vi "main.vi"() -> ()   [LabVIEW 2009]
uses:
  subvi/activity_info.vi
  <vilib>/Utility/file.llb/Write To Spreadsheet File (DBL).vi
panel:
  in  "Slide":cluster{dbl, dbl}(slide) scale=0.0..1.0
  out "above threshold":dbl(slide) scale=0.0..1.0
  in  "Threshold":dbl(slide)=0.85 scale=0.0..1.0
  out "Correlations":dbl[](graph)
  out "Analyzing":u8(slide) scale=0.0..100.0
  in  "analyze correlations":bool
  in  "Reference Signal":i32
  in  "Reference Signals":dbl[][](array[numeric])
  in  "Save Signal":bool
  in  "read weights":bool
  out "max amplitude":dbl(slide) scale=0.0..2.0
  in  "Path":path=path "E:/Sensor/data/Craig walking ADI.csv"
  out "C":bool
  out "B":bool
  out "A":bool
  in  "write data":bool
  out "Fundamental frequency":dbl(slide) scale=0.0..6.0
  in  "Normalize":bool
  out "high":bool
  out "med":bool
  out "low":bool
  out "RMS":dbl(slide) scale=0.0..10.0
  in  "write to memory":bool
  out "activity output":u16(ring) items=["A", "B", "C", "D"]
  out "output":dbl[](array[slide]) scale=0.0..1.0
  in  "stop learning":bool
  out "Error (training)":dbl(graph)
  in  "Learning Rate":dbl(slide)=0.336734693877551 scale=0.0..1.0
  in  "Beta":dbl(slide)=1.0 scale=0.0..1.0
  in  "train":bool
  in  "Number of hidden neurons":i32(slide)=9 scale=0.0..20.0
  in  "delete state":bool
  in  "state":u32
  in  "activity":u16(ring) items=["A", "B", "C", "D", "E", "F", "G", "H"]
  in  "save state":bool
  in  "Tab Control":T1(tab)=enum."FFT on data 1"
  out "Time data on X',Y',Z'":T2(graph)
  out "FFT on X',Y',Z'":T3(graph)
  out "Filtered signal":dbl[](graph)
  out "Magnitude of time data":cluster{dbl[], dbl[]}(graph)
  out "activity states":T4(graph)
  in  "Sensor":u16(ring) items=["Sensor 1", "Sensor 2", "Sensor 3"]
  in  "Sensor Type":u16(ring) items=["Acceleration", "Rotation"]
  in  "Sensor Brand 1":u16(ring) items=["ADXL", "Kinetisense"]
  in  "End time (s) 1":dbl(slide)=10.0 scale=0.0..200.0
  in  "FFT interval (s) 1":dbl(slide)=4.0 scale=0.0..40.0
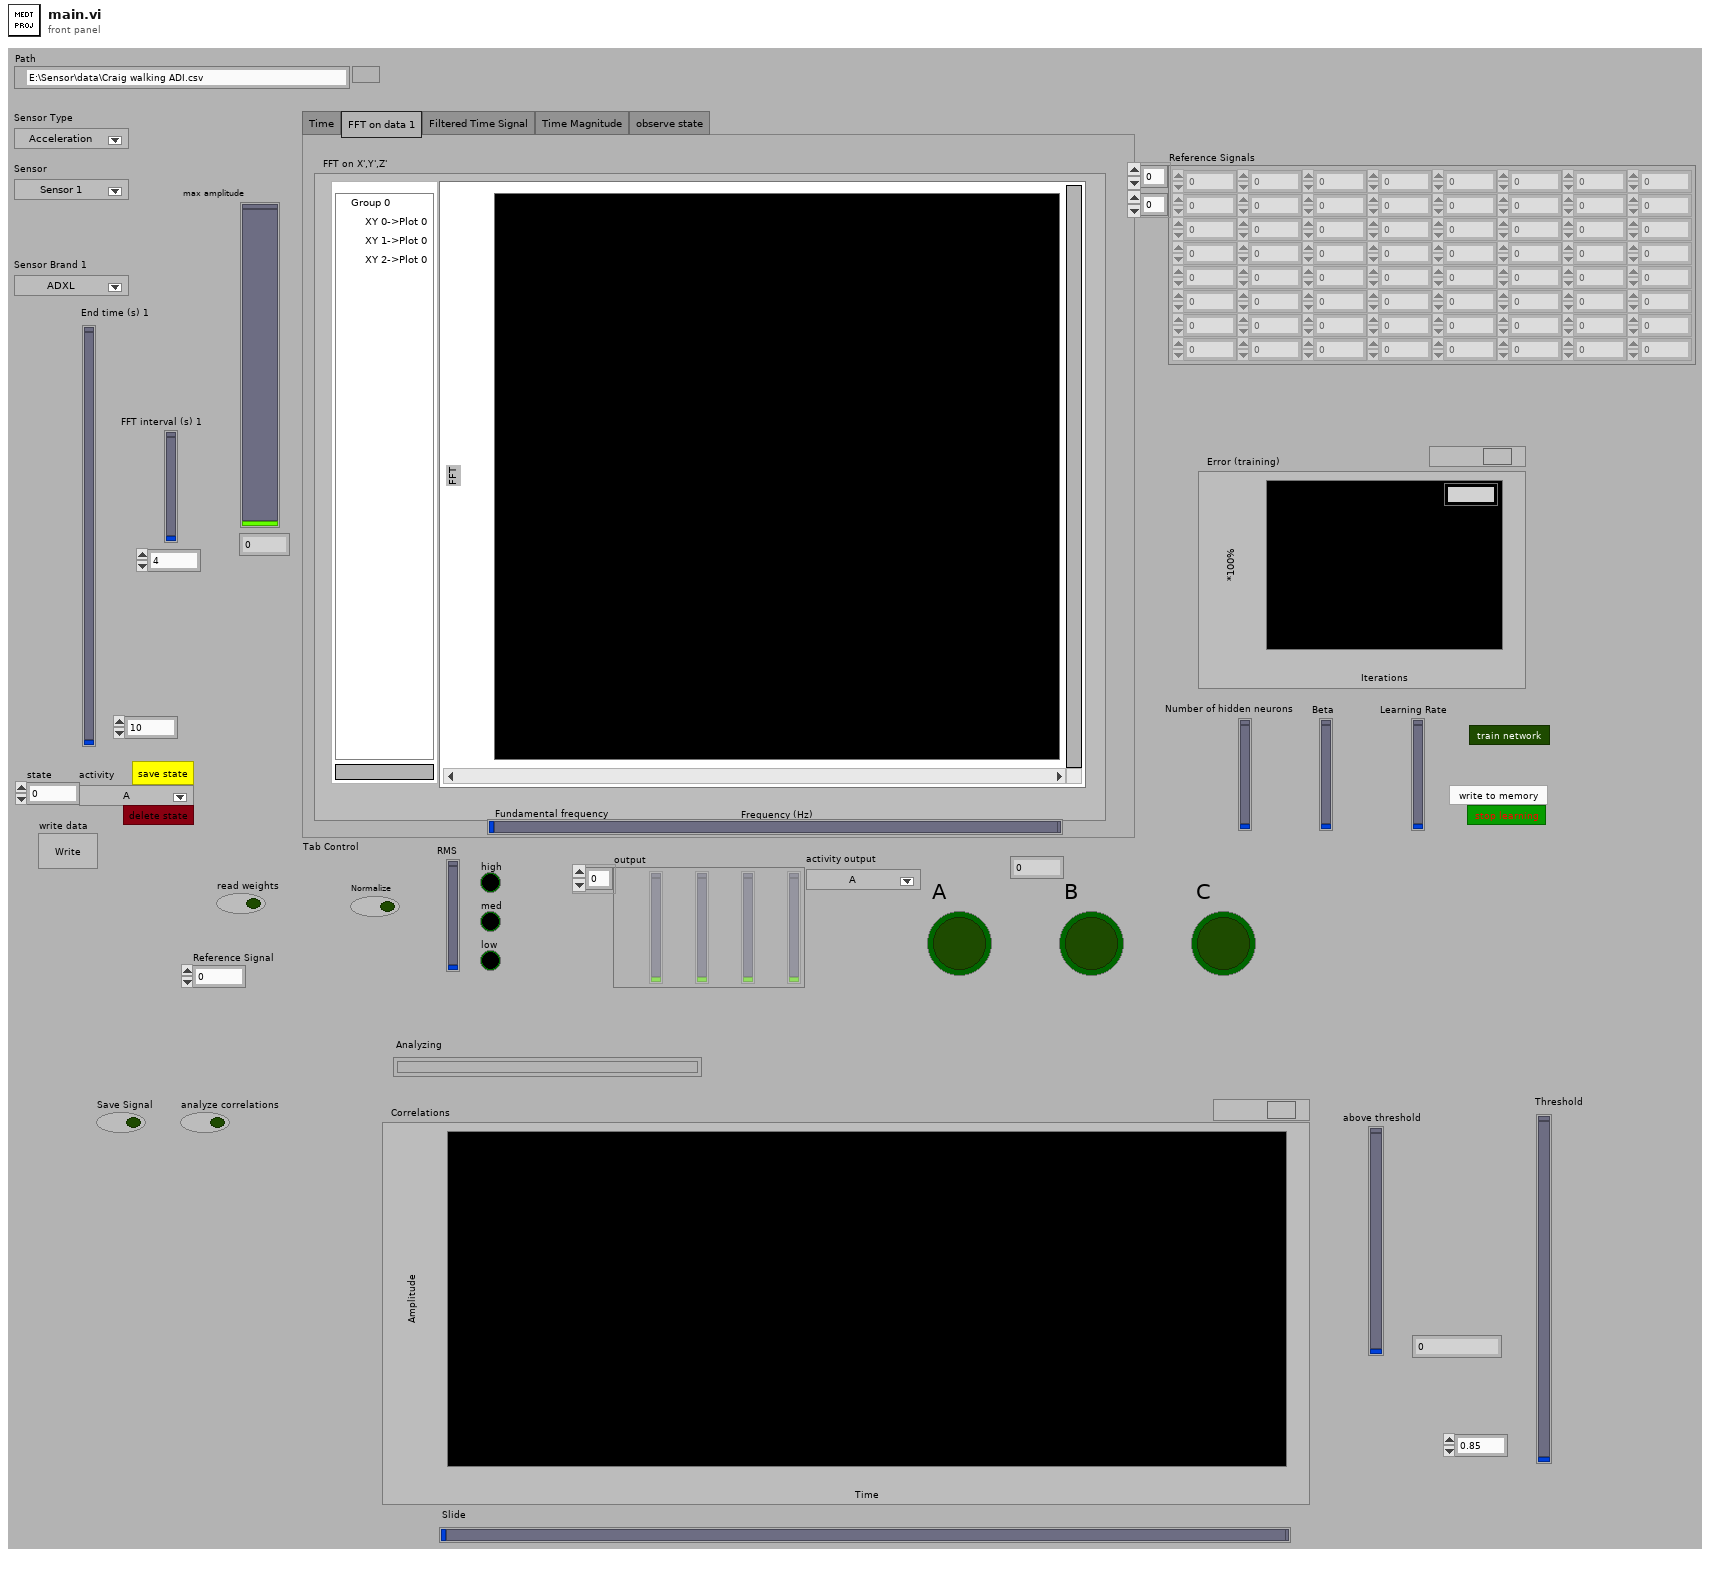
[diagram p1: front panel]
types:
  T1 = enum32{"Time", "FFT on data 1", "Filtered Time Signal", "Time Magnitude", "observe state"}
  T2 = cluster{cluster{dbl[], "Data out":dbl[]}, cluster{dbl[], "Data out":dbl[]}, cluster{dbl[], "Data out":dbl[]}}
  T3 = cluster{"XY Graph":cluster{dbl[], "magnitude":dbl[]}, "XY Graph":cluster{dbl[], "magnitude":dbl[]}, "XY Graph":cluster{dbl[], "magnitude":dbl[]}}
  T4 = cluster{cluster{dbl[], "Bicycling":dbl[]}, cluster{dbl[], "Bicycling":dbl[]}, cluster{dbl[], dbl[]}, cluster{dbl[], dbl[]}, cluster{dbl[], dbl[]}}
  T5 = cluster{"activity":u16, "save state":bool, "state":u32, bool, "peaks":dbl[][], bool}
  T6 = cluster{"activity":u16, "save state":bool, "state":u32, bool, "peaks":dbl[][], "write to memory":bool}
  T7 = cluster{"A":dbl[][], "B":dbl[][], "C":dbl[][], "D":dbl[][], "E":dbl[][], "F":dbl[][], "G":dbl[][], "H":dbl[][]}
  T8 = cluster{cluster{dbl[], dbl[]}, cluster{dbl[], dbl[]}, cluster{dbl[], dbl[]}}
  T9 = cluster{"Cluster":cluster{dbl[], "activity":dbl[]}, "Cluster":cluster{dbl[], "activity":dbl[]}, cluster{dbl[], dbl[]}, cluster{dbl[], dbl[]}, cluster{dbl[], dbl[]}}
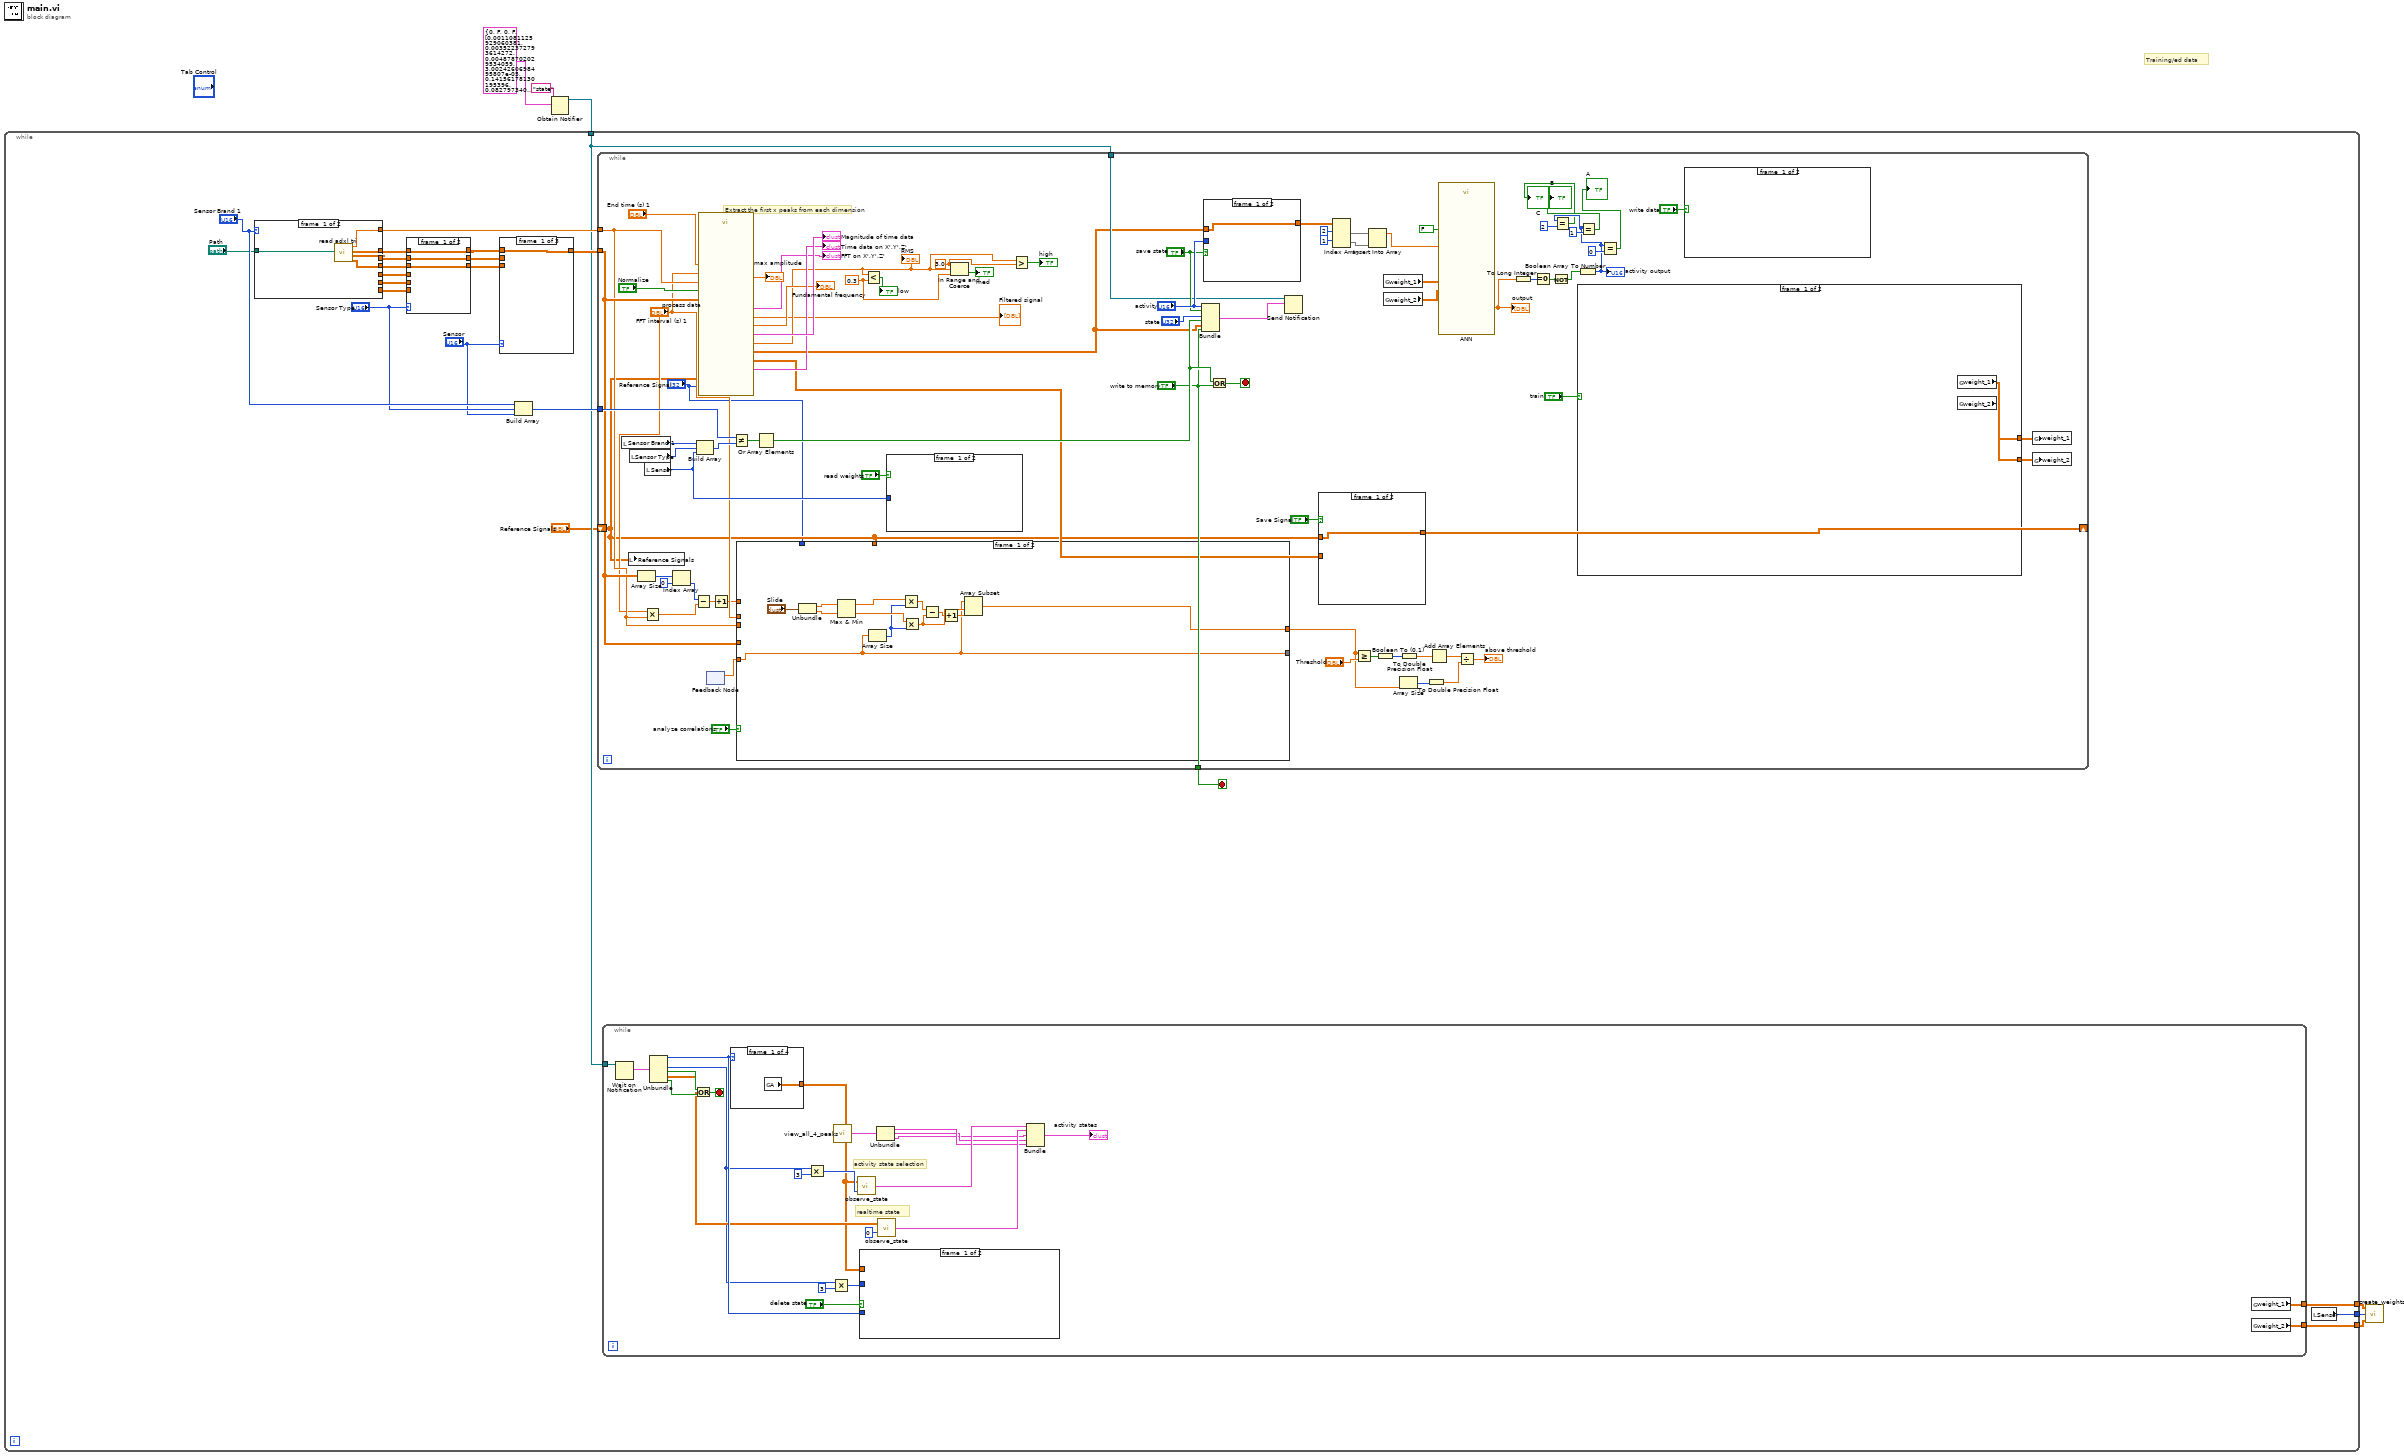
[diagram p0: block diagram]
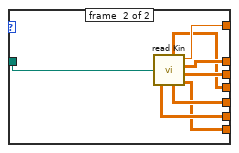
[diagram p5: hidden frame]
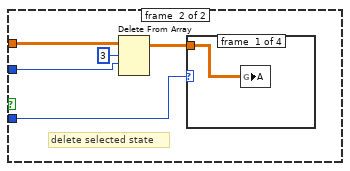
[diagram p6: hidden frame]
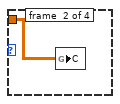
[diagram p7: hidden frame]
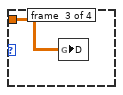
[diagram p8: hidden frame]
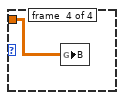
[diagram p9: hidden frame]
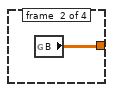
[diagram p10: hidden frame]
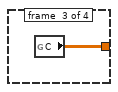
[diagram p11: hidden frame]
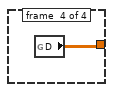
[diagram p12: hidden frame]
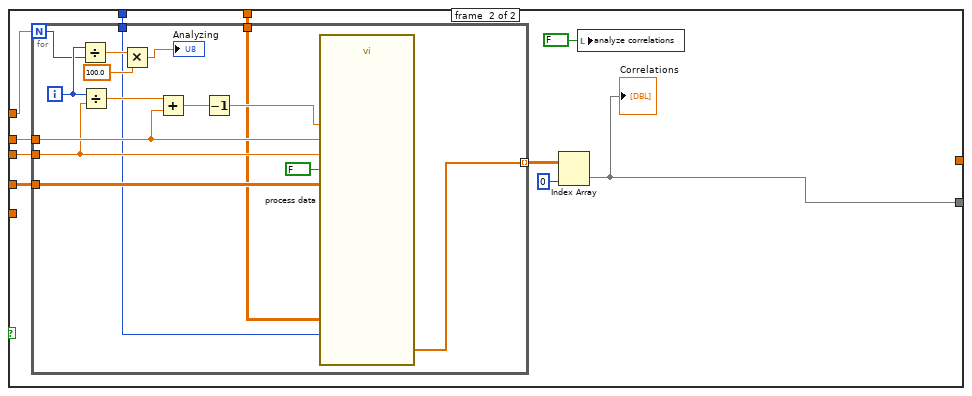
[diagram p13: hidden frame]
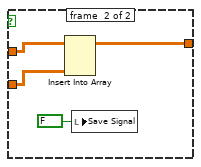
[diagram p14: hidden frame]
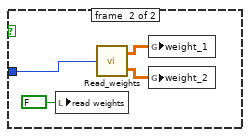
[diagram p15: hidden frame]
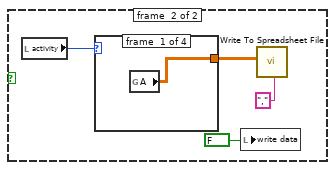
[diagram p16: hidden frame]
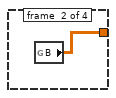
[diagram p17: hidden frame]
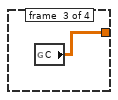
[diagram p18: hidden frame]
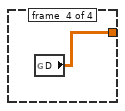
[diagram p19: hidden frame]
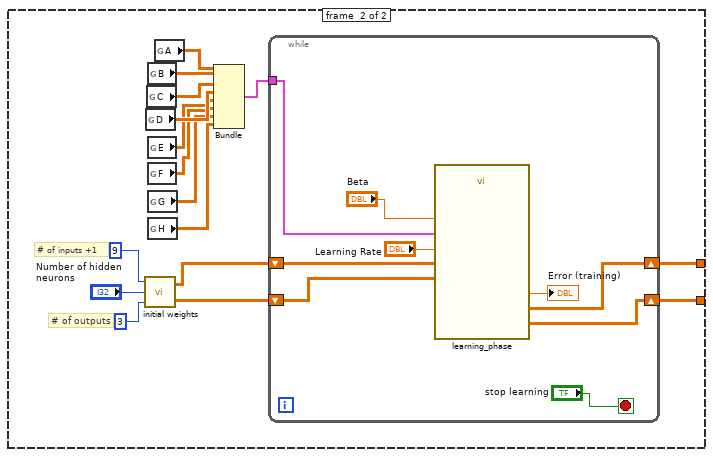
[diagram p20: hidden frame]
diagram:
  # "Training/ed data"
  n1 = Obtain Notifier(name (unnamed)="state", notification data type=T5 {"activity"=0, "save state"=FALSE, "state"=0, FALSE, "peaks"=[[0.0011081125929060381, 0.003522372793614272, 0.004878702029534059, 3.0024260698495807e-05], [0.14156178130195396, 0.08279734068484727, 0.022593374016756332, 0.00047669237690227347], [0.019524193753659796, 0.005914901850544118, 0.040958716531303056, 0.03788191680995928]], FALSE} ("output cluster")) -> (notifier out=w5:refnum<notifier>)  [unwired: 2 in, 2 out]
  n2 = while {
    tunnel: w5 -> [w25]
    tunnel: [w22] -> w3
    tunnel: [w21] -> w2
    tunnel: [w23] -> w1
    stop <- w24 stop-if-true
    n3 = case shown="0, Default" "Sensor Brand 1" {
      tunnel: [w42 w50] -> w28
      tunnel: [w41 w49] -> w19
      tunnel: [w40 w48] -> w20
      tunnel: [w39 w47] -> w18
      tunnel: [_ w46] -> w17
      tunnel: [_ w45] -> w16
      tunnel: [_ w44] -> w15
      tunnel: "Path" -> [w38 w43]
      frame #0 {
        n4 = call "read adxl tri.vi"("file path"=w38) -> ("sensor 3 acceleration"=w39:dbl[][], "sensor 2 acceleration"=w41:dbl[][], "sensor 1 acceleration"=w40:dbl[][], "Frequency (Hz)"=w42:dbl)  [unwired: 4 in]
      }
      frame #1 {
        n5 = call "read Kin.vi"("file path"=w43) -> ("sensor 3 rotation"=w44:dbl[][], "sensor 1 rotation"=w46:dbl[][], "sensor 2 acceleration"=w49:dbl[][], "sensor 1 acceleration"=w48:dbl[][], "sensor 3 acceleration"=w47:dbl[][], "Frequency (Hz)"=w50:dbl, "sensor 2 rotation"=w45:dbl[][])  [unwired: 1 in]
      }
    }
    n6 = case shown="0, Default" "Sensor Type" {
      tunnel: w20 -> [w34 _]
      tunnel: w19 -> [w33 _]
      tunnel: w18 -> [w32 _]
      tunnel: w17 -> [_ w37]
      tunnel: w16 -> [_ w36]
      tunnel: w15 -> [_ w35]
      tunnel: [w34 w37] -> w9
      tunnel: [w33 w36] -> w14
      tunnel: [w32 w35] -> w13
      frame #0 {
      }
      frame #1 {
      }
    }
    n7 = case shown="0, Default" "Sensor" {
      tunnel: w9 -> [w29 _ _]
      tunnel: w14 -> [_ w30 _]
      tunnel: w13 -> [_ _ w31]
      tunnel: [w29 w30 w31] -> w27
      frame #0 {
      }
      frame #1 {
      }
      frame #2 {
      }
    }
    n8 = Build Array("Sensor Brand 1", "Sensor Type", "Sensor") -> (w26:u16[])
    n9 = while {
      tunnel: w28 -> [w107]
      tunnel: w27 -> [w110]
      tunnel: w26 -> [w158]
      tunnel: w25 -> [w154]
      tunnel: ["write to memory"] -> w24
      shift-right: [w112] -> _
      shift-left: "Reference Signals" -> [w101]
      stop <- w135 stop-if-true
      w129 = 3.0 ("upper limit")
      w131 = 0.3 ("y")
      # "Extract the first x peaks from each dimension"
      n10 = local read "Sensor Brand 1"() -> (w162:u16)
      n11 = local write "Reference Signals"(w101) -> ()
      n12 = local read "Sensor Type"() -> (w161:u16)
      n13 = Array Size(array=w110) -> (size(s)=w109:i32[])
      n14 = Multiply(x="FFT interval (s) 1", y=w107) -> (x*y=w105:dbl)
      n15 = local read "Sensor"() -> (w115:u16)
      n16 = Index Array(array=w109, index=0) -> (element=w104:i32)
      n17 = Subtract(x=w104, y=w105) -> (x-y=w103:dbl)
      n18 = Build Array(w162, w161, w115) -> (w160:u16[])
      n19 = call "process data.vi"("Frequency (Hz)"=w107, "Reference Signal"="Reference Signal", "sensor input"=w110, "In Signals"=w101, "FFT interval (s)"="FFT interval (s) 1", "Normalize"="Normalize", "End time (s)"="End time (s) 1") -> ("Fundamental frequency"=→"Fundamental frequency":dbl, "FFT"=→"FFT on X',Y',Z'":T3, "peaks"=w134:dbl[][], "Magnitude of time data"=→"Magnitude of time data":cluster{dbl[], dbl[]}, "x',y',z'"=→"Time data on X',Y',Z'":T2, "Signals"=w111:dbl[][], "Filtered signal"=→"Filtered signal":dbl[], "max amplitude"=w117:dbl)  [unwired: 1 out]
      "RMS" <- w117
      "max amplitude" <- w117
      n20 = feedback #1() -> (w89:dbl[])  [unwired: 1 in]
      n21 = Increment(x=w103) -> (x+1=w102:dbl)
      n22 = Not Equal?(x=w158, y=w160) -> (x != y?=w159:bool[])
      n23 = case shown="False" "analyze correlations" {
        tunnel: w110 -> [_ w188]
        tunnel: w107 -> [_ w187]
        tunnel: "FFT interval (s) 1" -> [_ w186]
        tunnel: w102 -> [_ w185]
        tunnel: w101 -> [_ w184]
        tunnel: "Reference Signal" -> [_ w180]
        tunnel: [w168 w179] -> w90
        tunnel: w89 -> [w168 _]
        tunnel: [w167 _] -> w88
        frame #0 {
          n24 = Unbundle("Slide") -> (w177:dbl, w176:dbl)
          n25 = Max & Min(x=w177, y=w176) -> (max(x,y)=w173:dbl, min(x,y)=w175:dbl)
          n26 = Array Size(array=w168) -> (size(s)=w174:i32)
          n27 = Multiply(x=w173, y=w174) -> (x*y=w172:dbl)
          n28 = Multiply(x=w175, y=w174) -> (x*y=w171:dbl)
          n29 = Subtract(x=w172, y=w171) -> (x-y=w169:dbl)
          n30 = Increment(x=w169) -> (x+1=w170:dbl)
          n31 = Array Subset(array=w168, index=w171, length=w170) -> (w167:dbl[])
        }
        frame #1 {
          n32 = for {
            N: w185 -> [w193]
            tunnel: w188 -> [w202]
            tunnel: w186 -> [w200]
            tunnel: w187 -> [w199]
            tunnel: [w201] -> w182 mode=indexing
            tunnel: w184 -> [w195]
            tunnel: w180 -> [w189]
            i -> [w194]
            n33 = Divide(x=w194, y=w193) -> (x/y=w192:dbl)
            n34 = Divide(x=w194, y=w199) -> (x/y=w198:dbl)
            n35 = Multiply(x=w192, y=100.0) -> (x*y=→"Analyzing":dbl)
            n36 = Add(x=w198, y=w200) -> (x+y=w197:dbl)
            n37 = Decrement(x=w197) -> (x-1=w196:dbl)
            n38 = call "process data.vi"("Frequency (Hz)"=w199, "Reference Signal"=w189, "sensor input"=w202, "In Signals"=w195, "FFT interval (s)"=w200, "Normalize"=FALSE, "End time (s)"=w196) -> ("correlation array"=w201:dbl[])  [unwired: 8 out]
          }
          n39 = Index Array(array=w182, index (col)=0 ("disabled index (col)")) -> (element=w179:dbl[])  [unwired: 1 in]
          "Correlations" <- w179
          n40 = local write "analyze correlations"(FALSE ("analyze correlations")) -> ()
        }
      }
      n41 = Or Array Elements(Boolean array=w159) -> (logical OR=w136:bool)
      n42 = Less?(x=w117, y=w131) -> (x < y?=→"low":bool)
      n43 = case shown="True" "read weights" {
        tunnel: w115 -> [_ w212]
        frame #0 {
        }
        frame #1 {
          n44 = local write "read weights"(FALSE ("read weights")) -> ()
          n45 = call "Read_weights.vi"("sensor"=w212) -> ("weights 1"=w210:dbl[][], "weights 2"=w209:dbl[][])
          n46 = global write "activity_info.vi" "weight_1"(w210) -> ()
          n47 = global write "activity_info.vi" "weight_2"(w209) -> ()
        }
      }
      n48 = In Range and Coerce(upper limit=w129, x=w117, lower limit=w131) -> (In Range?=→"med":bool)  [unwired: 1 out]
      n49 = Greater?(x=w117, y=w129) -> (0:→"high":bool)
      n50 = Bundle("activity"="activity", "save state"="save state", "state"="state", w136, "peaks"=w134, "write to memory"="write to memory") -> (w153:T6)  [unwired: 1 in]
      n51 = case shown="True" "save state" {
        tunnel: w134 -> [w248 w250]
        tunnel: [w248 w250] -> w146
        tunnel: "activity" -> [_ w249]
        frame #0 {
        }
        frame #1 {
          # "save the state to  temp memory"
          n52 = call "save_state.vi"("state"=w249, "peaks"=w250) -> ()  [unwired: 1 in]
        }
      }
      n53 = Or(x=w136, y="write to memory") -> (x .or. y?=w135:bool)
      n54 = Send Notification(notification=w153, notifier=w154) -> ()  [unwired: 1 in, 2 out]
      n55 = case shown="True" "Save Signal" {
        tunnel: w111 -> [_ w208]
        tunnel: [w204 w205] -> w112
        tunnel: w101 -> [w204 w206]
        frame #0 {
        }
        frame #1 {
          n56 = Insert Into Array(array=w206, new element=w208) -> (w205:dbl[][])  [unwired: 2 in]
          n57 = local write "Save Signal"(FALSE ("Save Signal")) -> ()
        }
      }
      n58 = Index Array(array=w146, index (row) #1=2 ("index (row)"), index (row) #2=1 ("index (row)")) -> (element #1=w149:dbl[], element #2=w148:dbl[])  [unwired: 2 in]
      n59 = Greater Or Equal?(x=w88, y="Threshold") -> (x >= y?=w92:bool[])
      n60 = Insert Into Array(array=w149, new element=w148) -> (w147:dbl[])  [unwired: 1 in]
      n61 = Boolean To (0,1)(Boolean=w92) -> (0, 1=w93:i16[])
      n62 = global read "activity_info.vi" "weight_1"() -> (w145:dbl[][])
      n63 = global read "activity_info.vi" "weight_2"() -> (w144:dbl[][])
      n64 = Array Size(array=w88) -> (size(s)=w96:i32)
      n65 = To Double Precision Float(number=w93) -> (double precision float=w94:dbl[])
      n66 = To Double Precision Float(number=w96) -> (double precision float=w97:dbl)
      n67 = Add Array Elements(numeric array=w94) -> (sum=w95:dbl)
      n68 = call "ANN.vi"("Input"=w147, "Weight_2"=w144, "Weight_1"=w145, "Back Propagation"=FALSE) -> ("output"=w140:dbl[])  [unwired: 8 in, 3 out]
      "output" <- w140
      n69 = Divide(x=w95, y=w97) -> (x/y=→"above threshold":dbl)
      n70 = To Long Integer(number=w140) -> (32bit integer=w139:i32[])
      n71 = Equal To 0?(x=w139) -> (x = 0?=w138:bool[])
      n72 = Not(x=w138) -> (.not. x?=w137:bool[])
      n73 = case shown="True" "train" {
        tunnel: [w221 w230] -> w143
        tunnel: [w222 w229] -> w142
        frame #0 {
          n74 = global read "activity_info.vi" "weight_1"() -> (w222:dbl[][])
          n75 = global read "activity_info.vi" "weight_2"() -> (w221:dbl[][])
        }
        frame #1 {
          # "# of inputs +1"
          # "# of outputs"
          n76 = call "initial weights.vi"("Number of classifiers"=3, "Number of hidden neurons"="Number of hidden neurons", "Inputs + 1"=9) -> ("Weights 2"=w238:dbl[][], "Weights 1"=w237:dbl[][])
          n77 = global read "activity_info.vi" "D"() -> (w231:dbl[][])
          n78 = global read "activity_info.vi" "C"() -> (w235:dbl[][])
          n79 = global read "activity_info.vi" "B"() -> (w234:dbl[][])
          n80 = global read "activity_info.vi" "E"() -> (w226:dbl[][])
          n81 = global read "activity_info.vi" "F"() -> (w225:dbl[][])
          n82 = global read "activity_info.vi" "G"() -> (w224:dbl[][])
          n83 = global read "activity_info.vi" "H"() -> (w223:dbl[][])
          n84 = global read "activity_info.vi" "A"() -> (w228:dbl[][])
          n85 = Bundle("A"=w228, "B"=w234, "C"=w235, "D"=w231, "E"=w226, "F"=w225, "G"=w224, "H"=w223) -> (w236:T7)  [unwired: 1 in]
          n86 = while {
            tunnel: w236 -> [w247]
            shift-right: [w244] -> w229
            shift-left: w237 -> [w246]
            shift-right: [w243] -> w230
            shift-left: w238 -> [w245]
            stop <- "stop learning" stop-if-true
            n87 = call "learning_phase.vi"("Weights 2"=w245, "Weights 1"=w246, "Learning Rate"="Learning Rate", "Beta"="Beta", "inputs"=w247) -> ("Error"=→"Error (training)":dbl, "Weight_2_out"=w243:dbl[][], "Weight_1_out"=w244:dbl[][])
          }
        }
      }
      n88 = Boolean Array To Number(Boolean array=w137) -> (number=w120:u32)
      "activity output" <- w120
      n89 = Equal?(x=w120, y=u32 2) -> (x = y?=→"C":bool)
      n90 = Equal?(x=w120, y=u32 1) -> (x = y?=→"B":bool)
      n91 = Equal?(x=w120, y=u32 0) -> (x = y?=→"A":bool)
      n92 = case shown="True" "write data" {
        frame #0 {
        }
        frame #1 {
          n93 = local read "activity"() -> (w216:u16)
          n94 = case shown="0, Default" w216 {
            tunnel: [w217 w218 w219 w220] -> w215
            frame #0 {
              n95 = global read "activity_info.vi" "A"() -> (w217:dbl[][])
            }
            frame #1 {
              n96 = global read "activity_info.vi" "B"() -> (w218:dbl[][])
            }
            frame #2 {
              n97 = global read "activity_info.vi" "C"() -> (w219:dbl[][])
            }
            frame #3 {
              n98 = global read "activity_info.vi" "D"() -> (w220:dbl[][])
            }
          }
          n99 = local write "write data"(FALSE ("write data")) -> ()
          n100 = call-poly <vilib>:"Write To Spreadsheet File.vi"("delimiter (\\t)"="," ("delimiter (\\t)"), "2D data"=w215) -> ()  [unwired: 6 in, 1 out]
        }
      }
      n101 = global write "activity_info.vi" "weight_1"(w142) -> ()
      n102 = global write "activity_info.vi" "weight_2"(w143) -> ()
    }
    n103 = while {
      tunnel: w25 -> [w74]
      tunnel: [w63] -> w22
      tunnel: [w62] -> w21
      stop <- w66 stop-if-true
      # "activity state selection"
      # "realtime state"
      n104 = Wait on Notification(notifier=w74) -> (notification=w73:T5)  [unwired: 3 in, 3 out]
      n105 = Unbundle(w73) -> ("activity"=w69:u16, "state"=w51:u32, w67:bool, "peaks"=w59:dbl[][], w64:bool)  [unwired: 1 out]
      n106 = Or(x=w67, y=w64) -> (x .or. y?=w66:bool)
      n107 = case shown="3" w69 {
        tunnel: [w84 w85 w86 w87] -> w52
        frame #0 {
          n108 = global read "activity_info.vi" "A"() -> (w84:dbl[][])
        }
        frame #1 {
          n109 = global read "activity_info.vi" "B"() -> (w85:dbl[][])
        }
        frame #2 {
          n110 = global read "activity_info.vi" "C"() -> (w86:dbl[][])
        }
        frame #3 {
          n111 = global read "activity_info.vi" "D"() -> (w87:dbl[][])
        }
      }
      n112 = Multiply(x=w51, y=u32 3) -> (x*y=w70:u32)
      n113 = Multiply(x=w51, y=u32 3) -> (x*y=w60:u32)
      n114 = call "view_all_4_peaks.vi"("activity"=w52) -> ("Cluster"=w56:T8)
      n115 = call "observe_state.vi"("Numeric"=w70, "activity"=w52) -> ("Cluster"=w68:cluster{dbl[], "activity":dbl[]})
      n116 = case shown="True" "delete state" {
        tunnel: w52 -> [_ w79]
        tunnel: w60 -> [_ w77]
        tunnel: w69 -> [_ w76]
        frame #0 {
        }
        frame #1 {
          # "delete selected state"
          n117 = Delete From Array(array=w79, length=3, index (row)=w77) -> (array with subset deleted=w75:dbl[][])  [unwired: 1 in, 1 out]
          n118 = case shown="3" w76 {
            tunnel: w75 -> [w80 w81 w82 w83]
            frame #0 {
              n119 = global write "activity_info.vi" "A"(w80) -> ()
            }
            frame #1 {
              n120 = global write "activity_info.vi" "C"(w81) -> ()
            }
            frame #2 {
              n121 = global write "activity_info.vi" "D"(w82) -> ()
            }
            frame #3 {
              n122 = global write "activity_info.vi" "B"(w83) -> ()
            }
          }
        }
      }
      n123 = Unbundle(w56) -> (w55:cluster{dbl[], dbl[]}, w54:cluster{dbl[], dbl[]}, w53:cluster{dbl[], dbl[]})
      n124 = call "observe_state.vi"("Numeric"=u32 0, "activity"=w59) -> ("Cluster"=w57:cluster{dbl[], "activity":dbl[]})
      n125 = Bundle("Cluster"=w68, "Cluster"=w57, w53, w54, w55) -> (→"activity states":T9)  [unwired: 1 in]
      n126 = global read "activity_info.vi" "weight_1"() -> (w63:dbl[][])
      n127 = global read "activity_info.vi" "weight_2"() -> (w62:dbl[][])
    }
    n128 = local read "Sensor"() -> (w23:u16)
  }
  n129 = call "create_weights.vi"("weight2"=w2, "Ring"=w1, "weight1"=w3) -> ()
